vi "S2C_VAR_Globals.vi"() -> ()   [LabVIEW 2015]
panel:
  out "CurData":string[][](array[string])
  out "OrgData":string[][](array[string])
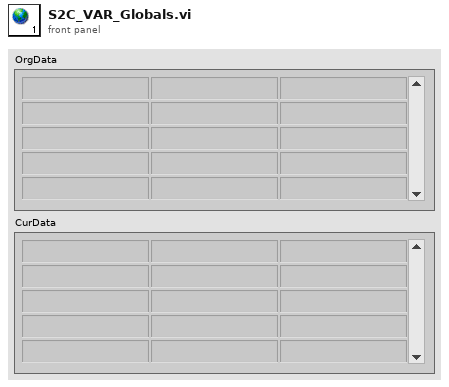
[diagram p1: front panel]
diagram:
